vi "GetSafetyStatus.vi"(10 "Ftp":refnum<k24>, 11 "error in":errorcluster) -> (2 "SafetyStatus":T1, 3 "error out":errorcluster)   [LabVIEW 2021, in "UnderAutomation.Fanuc.lvlib"]
uses:
  UnderAutomation.Fanuc.lvlib
  C:/Users/fg/Documents/Fanuc.vi/LabVIEW_2024/UnderAutomation.Fanuc/lib/UnderAutomation.Fanuc.dll
  LabVIEW_2024/UnderAutomation.Fanuc/lib/UnderAutomation.Fanuc.dll
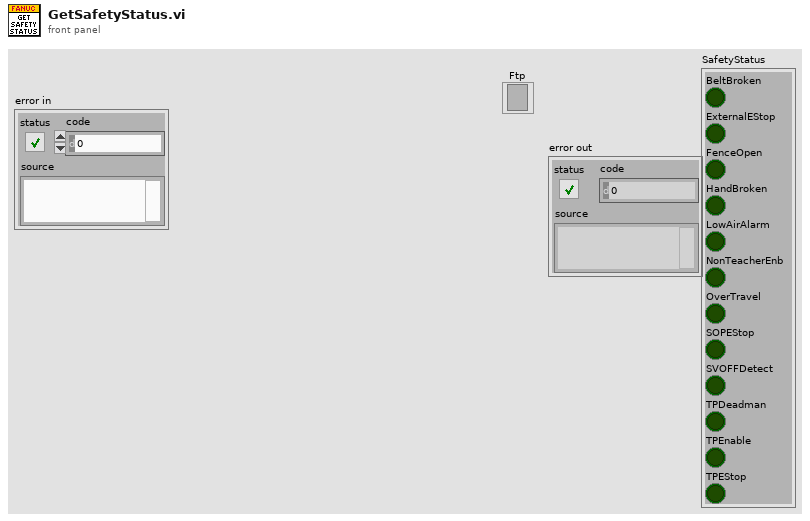
[diagram p1: front panel]
types:
  T1 = cluster{"BeltBroken":bool, "ExternalEStop":bool, "FenceOpen":bool, "HandBroken":bool, "LowAirAlarm":bool, "NonTeacherEnb":bool, "OverTravel":bool, "SOPEStop":bool, "SVOFFDetect":bool, "TPDeadman":bool, "TPEnable":bool, "TPEStop":bool}
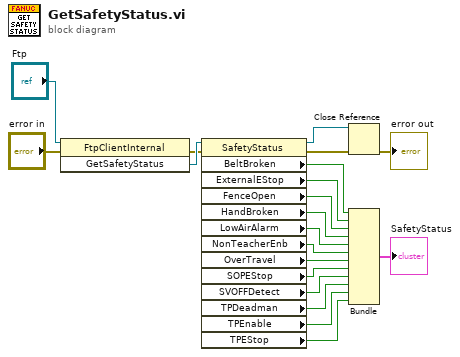
[diagram p0: block diagram]
diagram:
  n1 = invoke class="FtpClientInternal" method="GetSafetyStatus"(reference="Ftp", error in="error in") -> (error out=w17:errorcluster, "GetSafetyStatus"=w18:refnum<k24>)  [unwired: 1 in, 1 out]
  n2 = property class="SafetyStatus"(reference=w18, error in=w17) -> (reference out=w3:refnum<k24>, error out=w2:errorcluster, "BeltBroken"=w16:bool, "ExternalEStop"=w15:bool, "FenceOpen"=w14:bool, "HandBroken"=w13:bool, "LowAirAlarm"=w12:bool, "NonTeacherEnb"=w11:bool, "OverTravel"=w10:bool, "SOPEStop"=w9:bool, "SVOFFDetect"=w8:bool, "TPDeadman"=w7:bool, "TPEnable"=w6:bool, "TPEStop"=w5:bool)
  n3 = Close Reference(reference=w3, error in (no error)=w2) -> (error out=→"error out":errorcluster)
  n4 = Bundle("BeltBroken"=w16, "ExternalEStop"=w15, "FenceOpen"=w14, "HandBroken"=w13, "LowAirAlarm"=w12, "NonTeacherEnb"=w11, "OverTravel"=w10, "SOPEStop"=w9, "SVOFFDetect"=w8, "TPDeadman"=w7, "TPEnable"=w6, "TPEStop"=w5) -> (→"SafetyStatus":T1)  [unwired: 1 in]
